vi "OpenSpectraWiz.vi"(8 "error in (no error)":errorcluster, 11 "Microscope in":refnum<class "Microscope.lvclass">) -> (0 "error out":errorcluster, 3 "Microscope out":refnum<class "Microscope.lvclass">)   [LabVIEW 2012, in "Microscope.lvclass"]
uses:
  classes/Microscope.lvclass
  classes/Microscope.lvclass/Microscope.ctl
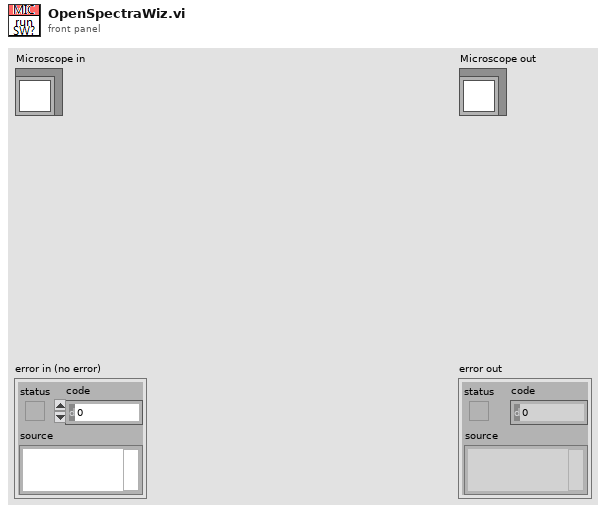
[diagram p1: front panel]
types:
  T1 = enum32{"Invalid", "Standard", "Closed", "Hidden", "Minimized", "Maximized"}
  T2 = typedef "DetectorType.ctl" = enum16{"PMT", "SpectraWiz"}
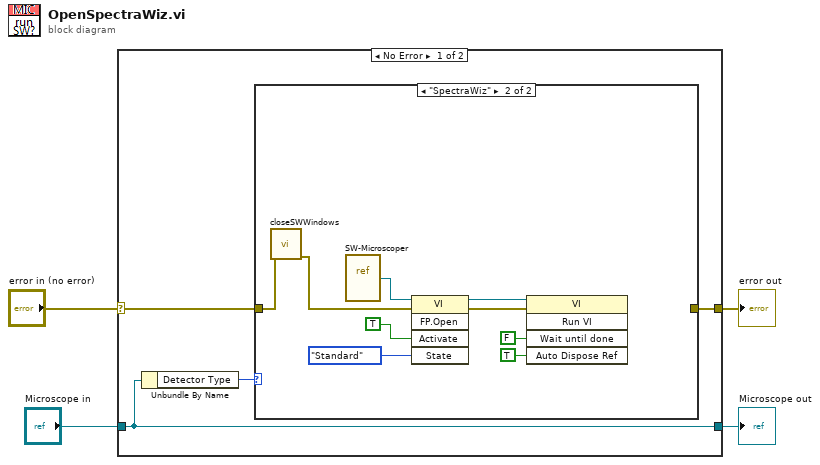
[diagram p0: block diagram]
diagram:
  n1 = case shown="No Error" "error in (no error)" {
    selector: "error in (no error)" -> [w6 w20]
    tunnel: [w5 w20] -> w3
    tunnel: [w8 w19] -> w1
    tunnel: "Microscope in" -> [w8 w19]
    frame No Error {
      n2 = Unbundle By Name(w8) -> ("Detector Type"=w7:T2)
      n3 = case shown="\"SpectraWiz\"" w7 {
        tunnel: [w9 _] -> w5
        tunnel: w6 -> [w9 w11]
        frame "PMT", Default {
        }
        frame "SpectraWiz" {
          n4 = call "closeSWWindows.vi"("error in (no error)"=w11) -> ("error out"=w10:errorcluster)  [unwired: 10 in]
          n5 = vi-ref "SW-Microscoper.vi"() -> (w15:refnum<vi>)
          n6 = invoke class="VI" method="FP.Open"(reference=w15, error in=w10, "Activate"=TRUE ("Activate?"), "State"=T1."Standard") -> (reference out=w16:refnum<vi>, error out=w13:errorcluster)  [unwired: 1 in, 3 out]
          n7 = invoke class="VI" method="Run VI"(reference=w16, error in=w13, "Wait until done"=FALSE ("Wait Until Done"), "Auto Dispose Ref"=TRUE ("Auto Dispose Reference")) -> ()  [unwired: 1 in, 5 out]
        }
      }
    }
    frame Error {
    }
  }
  "error out" <- w3
  "Microscope out" <- w1
